vi "Validate SLSC CD Reference.vi"(8 "error in":errorcluster, 11 "slsc switch custom device in":T1 format="%.0x") -> (0 "error out":errorcluster, 3 "slsc switch custom device out":T1 format="%.0x")   [LabVIEW 2020, in "SLSC Switch Scripting.lvlib"]
uses:
  SLSC Switch Scripting.lvlib
  <vilib>/NI VeriStand/Custom Device API/Custom Device Item Ref.ctl
  Shared/Constants.vi
  Dependencies.llb/SLSC Switch Shared.lvlib
  <vilib>/NI VeriStand/Custom Device API/Custom Device API.lvlib
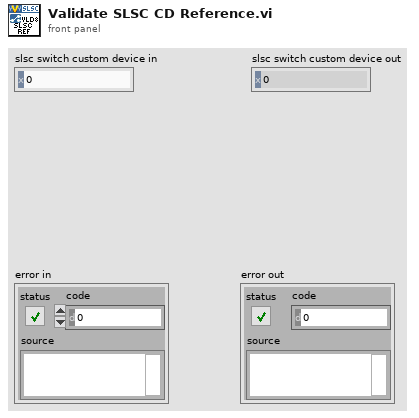
[diagram p1: front panel]
types:
  T1 = typedef "Custom Device API.lvlib/Custom Device Item Ref.ctl" = u64
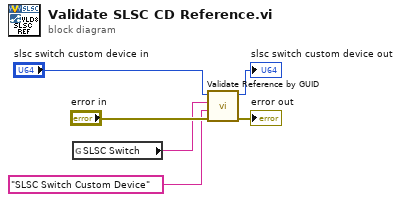
[diagram p0: block diagram]
diagram:
  n1 = global read "Constants.vi" "SLSC Switch"() -> (w1:string)
  n2 = call "Validate Reference by GUID.vi"("error in"="error in", "name"="SLSC Switch Custom Device" ("Name"), "guid"=w1, "slsc switch item in"="slsc switch custom device in") -> ("error out"=→"error out":errorcluster, "slsc switch item out"=→"slsc switch custom device out":T1)  [unwired: 6 in]
